vi "nirviRandomDataMultiElementFPGAFIFO.vi"(0 "Method":T1, 1 "Fifo":T2={"displayName"="", "hardwareName"="", "dataType"=enum."I16", "elementTypeDescriptor"=variant, "terminalTypeDescriptor"=variant, "requestedNumberOfElements"=2, "memoryType"=enum."Look-Up Table", "arbitrationForInterfaceA"=enum."Arbitrate if Multiple Requestors Only", "numberOfElementsPerRead"=1, "arbitrationForInterfaceB"=enum."Always Arbitrate", "numberOfElementsPerWrite"=1, "VI_Defined"=FALSE, "type"=enum."Target-Scoped", "initializationParameters"={"initialized"=FALSE, "VI_Path"=path "", "initialData"=variant}, "disableOnOverflow/Underflow"=FALSE, "interfaceConfiguration"=enum."Read A-Write B", "controlLogic"=enum."Slice Fabric", "actualNumberOfElements"=1027, "dramSelection"="", "dramMaxOustandingRequests"=0, "dramIncludeByteEnables"=FALSE, "dramGrantTime"=0, "fullEmulation"=FALSE, "memoryInMultipleClockDomains"=FALSE, "memoryLatency"=1} {"memoryLatency" items=["0", "1", "2", "3"]}, 3 "element in":variant, 5 "error in (no error)":errorcluster, 7 "Element Datatype":i32, 8 "In SCTL":bool, 9 "Input Valid?":bool, 11 "Timeout (ms)":i32, 13 "Ready for Output?":bool) -> (14 "element out":variant, 15 "Timed out":bool, 16 "Ready for Input":bool, 17 "count":u32, 18 "Output Valid":bool, 19 "error out":errorcluster)   [LabVIEW 2017]
uses:
  <vilib>/rvi/DataTransferAndStorage/Container/Common/niFpgaContainerState.ctl
  <vilib>/rvi/DataTransferAndStorage/Container/Common/niFpgaDataTypeControl.ctl
  <vilib>/rvi/DataTransferAndStorage/Container/Common/niFpgaContainerImplementationControl.ctl
  <vilib>/rvi/DataTransferAndStorage/Container/Common/niFpgaContainerArbitrationOptionsControl.ctl
  <vilib>/rvi/DataTransferAndStorage/Container/Common/niFpgaTransferTypeControl.ctl
  <vilib>/rvi/DataTransferAndStorage/Container/Common/niFpgaContainerInitializationParameters.ctl
  <vilib>/rvi/Memory/Memory_Types/niFpgaMemoryInterfaceConfiguration.ctl
  <vilib>/rvi/FIFO/Fifo_Types/niFpgaFifoControlLogicControl.ctl
  <vilib>/rvi/DataTransferAndStorage/Container/Common/niFpgaContainerMemoryLatencyControl.ctl
  <vilib>/rvi/DataTransferAndStorage/Container/Common/niFpgaContainerMethod.ctl
  <vilib>/rvi/interface/RandomDataEmulation/nirviQueueStoreOperation.ctl
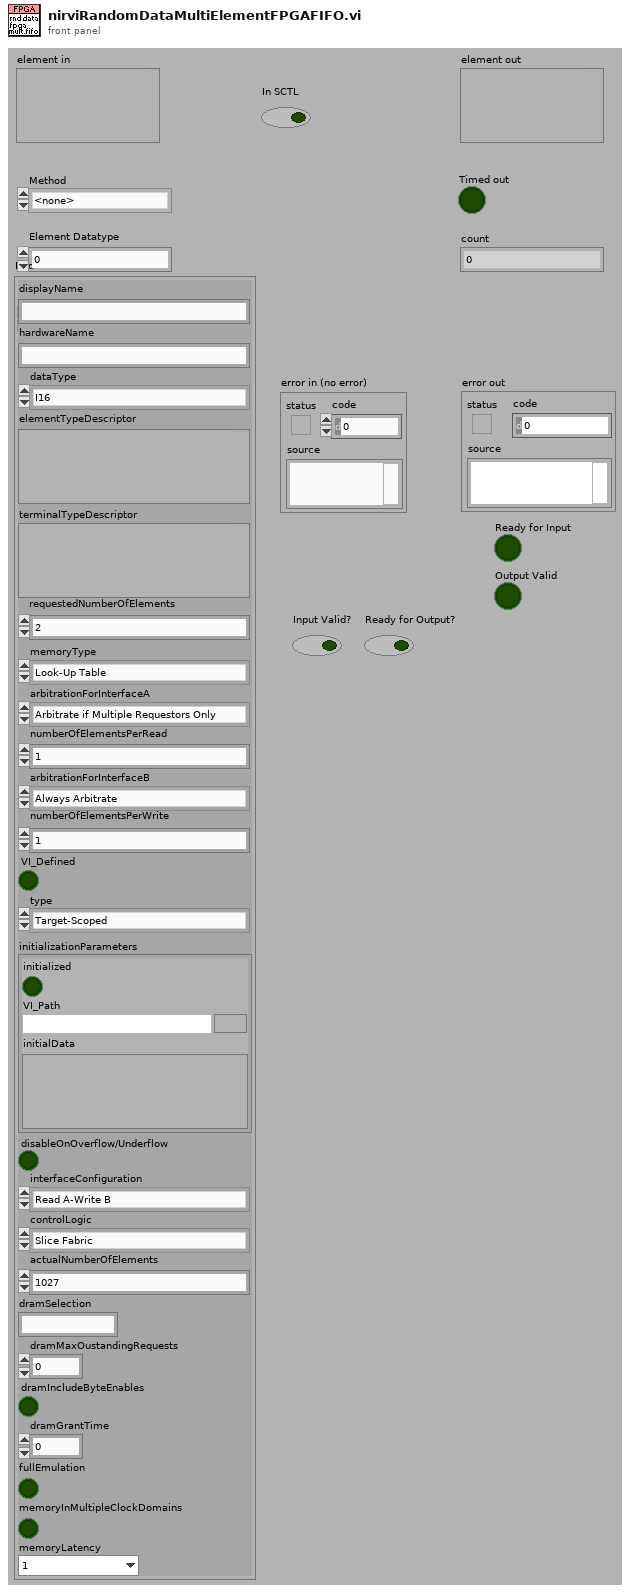
[diagram p1: front panel]
types:
  T1 = typedef "niFpgaContainerMethod.ctl" = enum16{"<none>", "write", "read", "clear", "getNumberOfElementsToWrite", "getNumberOfElementsToRead", "enable", "disable", "flushAndDisable", "getStreamState", "readA", "readB", "dramWrite", "dramWriteWithByteEnables", "dramRequestData", "dramRetrieveData", "readWithoutAcknowledge", "acknowledge", "writeUsingHandshaking", "readUsingHandshaking", "flush"}
  T2 = typedef "niFpgaContainerState.ctl" = cluster{"displayName":string, "hardwareName":string, "dataType":T3, "elementTypeDescriptor":variant, "terminalTypeDescriptor":variant, "requestedNumberOfElements":u32, "memoryType":T4, "arbitrationForInterfaceA":T5, "numberOfElementsPerRead":u32, "arbitrationForInterfaceB":T5, "numberOfElementsPerWrite":u32, "VI_Defined":bool, "type":T6, "initializationParameters":T7, "disableOnOverflow/Underflow":bool, "interfaceConfiguration":T8, "controlLogic":T9, "actualNumberOfElements":u32, "dramSelection":string, "dramMaxOustandingRequests":i32, "dramIncludeByteEnables":bool, "dramGrantTime":u32, "fullEmulation":bool, "memoryInMultipleClockDomains":bool, "memoryLatency":T10}
  T3 = typedef "niFpgaDataTypeControl.ctl" = enum32{"Boolean", "I8", "I16", "I32", "I64", "U8", "U16", "U32", "U64", "FXP", "CustomControl", "SGL"}
  T4 = typedef "niFpgaContainerImplementationControl.ctl" = enum16{"Flip-Flops", "Look-Up Table", "Block Memory", "DRAM"}
  T5 = typedef "niFpgaContainerArbitrationOptionsControl.ctl" = enum16{"Always Arbitrate", "Arbitrate if Multiple Requestors Only", "Never Arbitrate"}
  T6 = typedef "niFpgaTransferTypeControl.ctl" = enum16{"Target-Scoped", "Host to Target - DMA", "Target to Host - DMA", "Peer to Peer Reader", "Peer to Peer Writer", "Bidirectional"}
  T7 = typedef "niFpgaContainerInitializationParameters.ctl" = cluster{"initialized":bool, "VI_Path":path, "initialData":variant}
  T8 = typedef "niFpgaMemoryInterfaceConfiguration.ctl" = enum16{"Read A-Write B", "Read A-Read B"}
  T9 = typedef "niFpgaFifoControlLogicControl.ctl" = enum16{"Slice Fabric", "Target Optimal", "Built-in"}
  T10 = typedef "niFpgaContainerMemoryLatencyControl.ctl" = u16
  T11 = typedef "nirviQueueStoreOperation.ctl" = enum16{"Make New Queue", "Get Queue", "Resize Queue", "Close Queues", "Make New Lock", "Get Lock", "Get Host Fifo Size"}
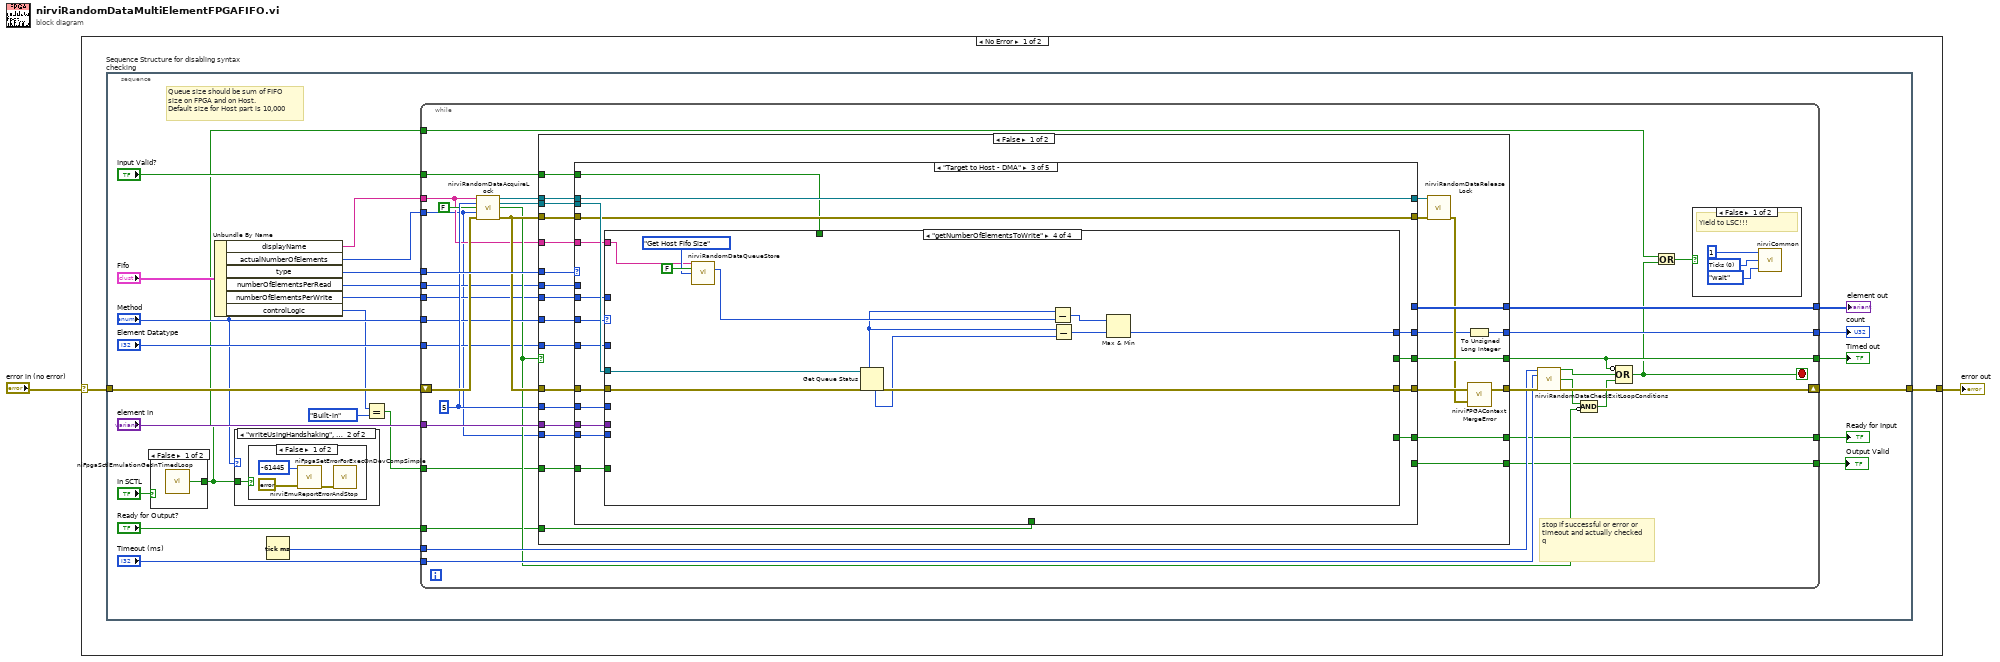
[diagram p0: block diagram]
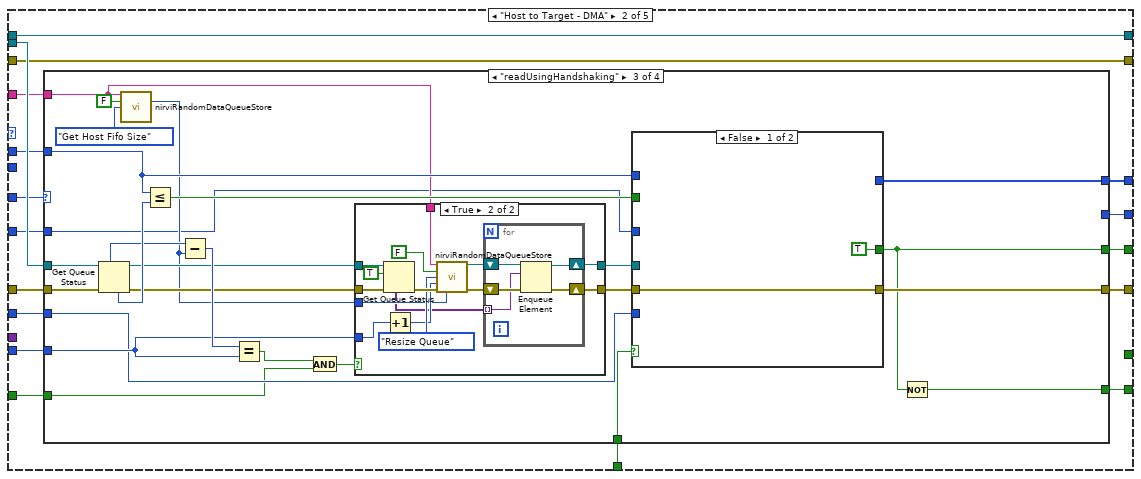
[diagram p7: hidden frame]
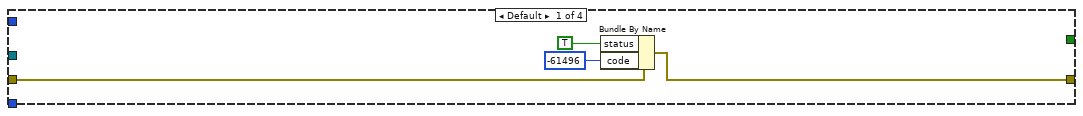
[diagram p8: hidden frame]
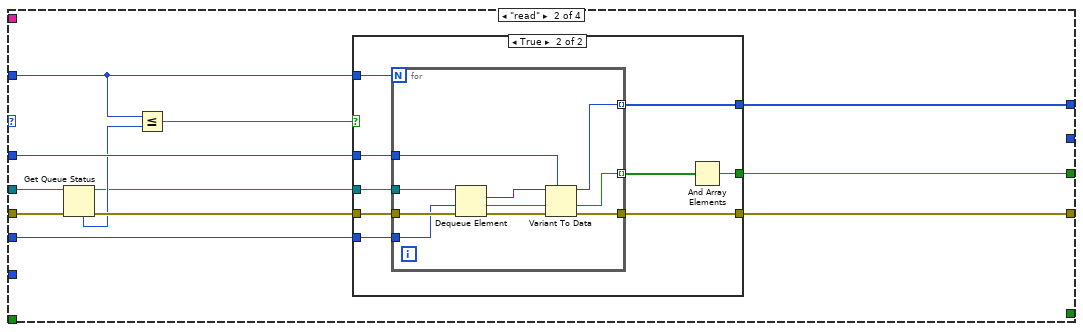
[diagram p9: hidden frame]
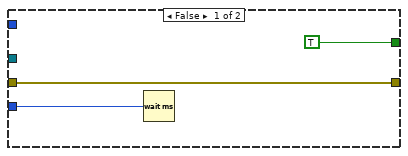
[diagram p10: hidden frame]
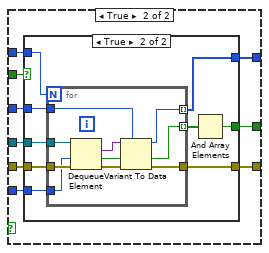
[diagram p11: hidden frame]
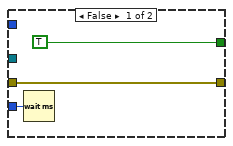
[diagram p12: hidden frame]
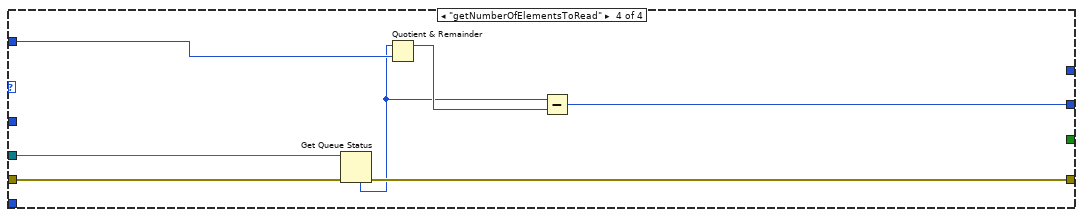
[diagram p14: hidden frame]
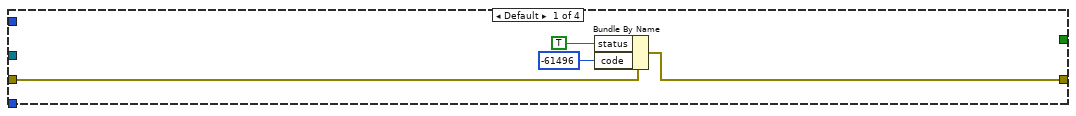
[diagram p15: hidden frame]
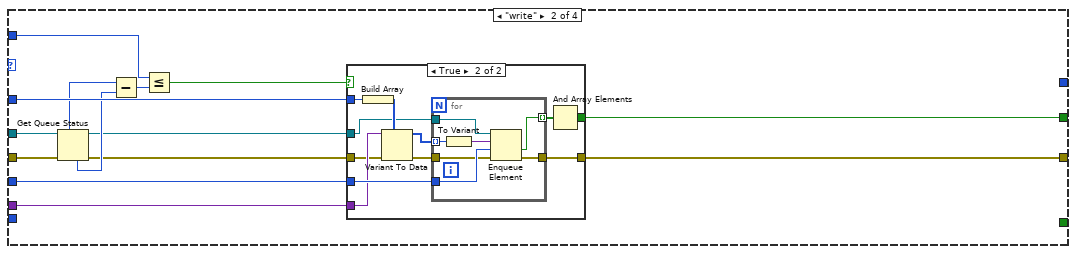
[diagram p16: hidden frame]
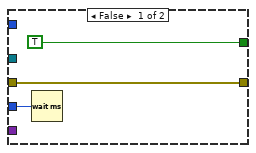
[diagram p17: hidden frame]
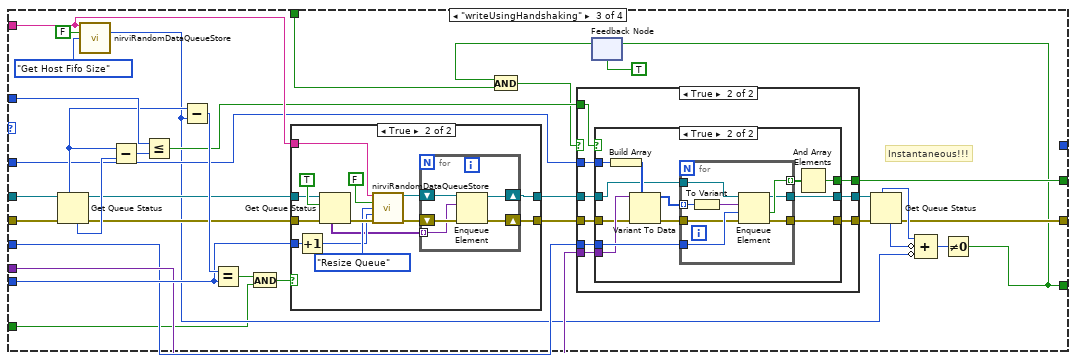
[diagram p18: hidden frame]
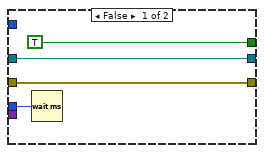
[diagram p20: hidden frame]
diagram:
  n1 = case shown="No Error" "error in (no error)" {
    selector: "error in (no error)" -> [w4 w413]
    tunnel: [w3 w413] -> w2
    frame No Error {
      n2 = stacked-sequence "Sequence Structure for disabling syntax checking" {
        tunnel: w4 -> [w15]
        tunnel: [w28] -> w3
        frame #0 {
          # "Queue size should be sum of FIFO\nsize on FPGA and on Host.\nDefault size for Host part is 10,000"
          n3 = case shown="False" "In SCTL" {
            selector: "In SCTL" -> [_ w31]
            tunnel: [w30 w31] -> w5
            frame False {
              n4 = call <vilib>:"niFpgaSctlEmulationGetInTimedLoop.vi"() -> ("x != 0?"=w30:bool)  [unwired: 15 in]
            }
            frame True {
            }
          }
          n5 = Unbundle By Name("Fifo") -> ("displayName"=w25:string, "actualNumberOfElements"=w23:u32, "type"=w22:T6, "numberOfElementsPerRead"=w18:u32, "numberOfElementsPerWrite"=w17:u32, "controlLogic"=w9:T9)
          n6 = case shown="\"writeUsingHandshaking\", \"readUsingHandshaking\"" "Method" {
            tunnel: w5 -> [_ w32]
            frame Default {
            }
            frame "writeUsingHandshaking", "readUsingHandshaking" {
              n7 = case shown="False" w32 {
                frame False {
                  n8 = call <vilib>:"niFpgaSetErrorForExecOnDevCompSimple.vi"("error code"=-61445, "error in"=errorcluster {"status"=FALSE, "code"=0, "source"=""}) -> ("error out"=w35:errorcluster)  [unwired: 13 in]
                  n9 = call <vilib>:"nirviEmuReportErrorAndStop.vi"("error to report"=w35) -> ()  [unwired: 1 in, 14 out]
                }
                frame True {
                }
              }
            }
          }
          n10 = Tick Count (ms)() -> (millisecond timer value=w27:u32)
          n11 = Equal?(x=w9, y=niFpgaFifoControlLogicControl."Built-in") -> (x = y?=w7:bool)
          n12 = while {
            tunnel: w22 -> [w66]
            tunnel: "element in" -> [w68]
            tunnel: "Timeout (ms)" -> [w62]
            tunnel: [w67] -> w26
            tunnel: [w54] -> w20
            tunnel: w27 -> [w63]
            tunnel: w25 -> [w45]
            shift-right: [w65] -> w28
            shift-left: w15 -> [w61]
            tunnel: w23 -> [w44]
            tunnel: "Method" -> [w55]
            tunnel: [w53] -> w19
            tunnel: "Element Datatype" -> [w48]
            tunnel: w18 -> [w47]
            tunnel: w17 -> [w46]
            tunnel: "Ready for Output?" -> [w43]
            tunnel: [w42] -> w12
            tunnel: "Input Valid?" -> [w41]
            tunnel: [w40] -> w10
            tunnel: w7 -> [w39]
            tunnel: w5 -> [w37]
            stop <- w38 stop-if-true
            w59 = 5 ("ms timeout (-1)")
            # "stop if successful or error or \ntimeout and actually checked q"
            n13 = call <vilib>:"nirviRandomDataAcquireLock.vi"("name"=w45, "ms timeout (-1)"=w59, "Host?"=FALSE, "fpga fifo size"=w44, "error in (no error)"=w61) -> ("lock out"=w60:refnum<queue>, "queue out"=w57:refnum<queue>, "timed out"=w52:bool, "error out"=w56:errorcluster)  [unwired: 7 out]
            n14 = case shown="False" w52 {
              selector: w52 -> [_ w412]
              tunnel: w68 -> [w84 _]
              tunnel: w59 -> [w98 _]
              tunnel: [w97 _] -> w67
              tunnel: [w93 w411] -> w64
              tunnel: [w96 w412] -> w54
              tunnel: w66 -> [w95 _]
              tunnel: w56 -> [w90 w411]
              tunnel: w60 -> [w85 _]
              tunnel: w57 -> [w91 _]
              tunnel: w56 -> [w88 _]
              tunnel: w55 -> [w87 _]
              tunnel: [w82 _] -> w53
              tunnel: w48 -> [w81 _]
              tunnel: w47 -> [w80 _]
              tunnel: w46 -> [w79 _]
              tunnel: w45 -> [w78 _]
              tunnel: w44 -> [w77 _]
              tunnel: w43 -> [w76 _]
              tunnel: [w75 _] -> w42
              tunnel: w41 -> [w74 _]
              tunnel: [w73 _] -> w40
              tunnel: w39 -> [w72 _]
              frame False {
                n15 = case shown="\"Target to Host - DMA\"" w95 {
                  tunnel: w98 -> [_ w117 w258 _ _]
                  tunnel: [_ w116 w256 _ _] -> w96
                  tunnel: [w101 w118 w259 w404 w405] -> w94
                  tunnel: [_ w108 _ _ _] -> w97
                  tunnel: w84 -> [_ _ w257 _ _]
                  tunnel: w90 -> [w101 w115 w255 w404 w406]
                  tunnel: w91 -> [_ w114 w254 _ _]
                  tunnel: [w100 w113 w253 w403 w407] -> w89
                  tunnel: w88 -> [w100 w113 w253 w403 w407]
                  tunnel: w87 -> [_ w111 w251 _ _]
                  tunnel: [w99 w112 w252 w402 w410] -> w86
                  tunnel: w85 -> [w99 w112 w252 w402 w410]
                  tunnel: [_ w110 w243 _ _] -> w83
                  tunnel: w81 -> [_ w109 w250 _ _]
                  tunnel: w80 -> [_ w107 _ _ _]
                  tunnel: w79 -> [_ _ w249 _ _]
                  tunnel: w78 -> [_ w106 w248 _ _]
                  tunnel: w77 -> [_ w105 w247 _ _]
                  tunnel: w76 -> [_ w104 _ _ _]
                  tunnel: [_ w103 _ _ _] -> w75
                  tunnel: w74 -> [_ _ w246 _ _]
                  tunnel: [_ _ w245 _ _] -> w73
                  tunnel: w72 -> [_ w102 w244 _ _]
                  frame "Target-Scoped" {
                    # "Not a DMA FIFO"
                  }
                  frame "Host to Target - DMA" {
                    n16 = case shown="\"readUsingHandshaking\"" w111 {
                      tunnel: [w119 w134 w181 w242] -> w118
                      tunnel: w117 -> [_ w132 w164 _]
                      tunnel: [_ w131 w161 _] -> w116
                      tunnel: w115 -> [w120 w129 w179 w240]
                      tunnel: w114 -> [_ w125 w176 w241]
                      tunnel: [_ _ _ w236] -> w110
                      tunnel: w109 -> [_ w133 w159 _]
                      tunnel: [_ w130 w180 _] -> w108
                      tunnel: w107 -> [_ w127 w178 w238]
                      tunnel: w106 -> [_ _ w170 _]
                      tunnel: w105 -> [_ _ w166 _]
                      tunnel: w104 -> [_ _ w162 _]
                      tunnel: [_ _ w160 _] -> w103
                      tunnel: w102 -> [_ _ w157 _]
                      frame Default {
                        n17 = Bundle By Name(cluster=w120, "status"=TRUE, "code"=-61496) -> (w119:errorcluster)
                      }
                      frame "read" {
                        n18 = Get Queue Status(queue=w125, error in (no error)=w129) -> (queue out=w124:refnum<queue>, error out=w128:errorcluster, # elements in queue=w126:i32)  [unwired: 1 in, 5 out]
                        n19 = Less Or Equal?(x=w127, y=w126) -> (x <= y?=w123:bool)
                        n20 = case shown="True" w123 {
                          tunnel: [w137 w146] -> w134
                          tunnel: w133 -> [_ w145]
                          tunnel: w132 -> [w135 w144]
                          tunnel: [TRUE ("timed out?") w138] -> w131
                          tunnel: [_ w143] -> w130
                          tunnel: w128 -> [w137 w142]
                          tunnel: w127 -> [_ w141]
                          tunnel: w124 -> [_ w140]
                          frame False {
                            n21 = Wait (ms)(milliseconds to wait=w135) -> ()  [unwired: 1 out]
                          }
                          frame True {
                            n22 = for {
                              N: w141 -> [_]
                              tunnel: [w155] -> w139 mode=indexing
                              tunnel: [w151] -> w146
                              tunnel: [w149] -> w143 mode=indexing
                              tunnel: w142 -> [w154]
                              tunnel: w145 -> [w150]
                              tunnel: w144 -> [w148]
                              tunnel: w140 -> [w147]
                              n23 = Dequeue Element(queue=w147, timeout in ms (-1)=w148, error in (no error)=w154) -> (element=w153:variant, timed out?=w155:bool, error out=w152:errorcluster)  [unwired: 1 out]
                              n24 = Variant To Data(error in=w152, type=w150, Variant=w153) -> (data=w149:i32, error out=w151:errorcluster)
                            }
                            n25 = And Array Elements(Boolean array=w139) -> (logical AND=w138:bool)
                          }
                        }
                      }
                      frame "readUsingHandshaking" {
                        n26 = Get Queue Status(queue=w176, error in (no error)=w179) -> (queue out=w169:refnum<queue>, max queue size=w172:i32, error out=w167:errorcluster, # elements in queue=w177:i32)  [unwired: 1 in, 4 out]
                        n27 = call <vilib>:"nirviRandomDataQueueStore.vi"("queue name"=w170, "Host?"=FALSE, "queue operation"=nirviQueueStoreOperation."Get Host Fifo Size") -> ("host fifo size out"=w165:u32)  [unwired: 9 in, 3 out]
                        n28 = Less Or Equal?(x=w178, y=w177) -> (x <= y?=w175:bool)
                        n29 = Subtract(x=w172, y=w165) -> (x-y=w171:u32)
                        n30 = Equal?(x=w171, y=w166) -> (x = y?=w158:bool)
                        n31 = And(x=w158, y=w157) -> (x .and. y?=w156:bool)
                        n32 = case shown="True" w156 {
                          tunnel: w167 -> [w214 w230]
                          tunnel: w169 -> [w215 w229]
                          tunnel: w170 -> [_ w226]
                          tunnel: w166 -> [_ w223]
                          tunnel: w165 -> [_ w221]
                          tunnel: [w215 w218] -> w168
                          tunnel: [w214 w216] -> w163
                          frame False {
                          }
                          frame True {
                            n33 = Get Queue Status(queue=w229, return elements? (F)=TRUE, error in (no error)=w230) -> (error out=w227:errorcluster, elements=w220:variant[])  [unwired: 6 out]
                            n34 = Increment(x=w223) -> (x+1=w222:u32)
                            n35 = call <vilib>:"nirviRandomDataQueueStore.vi"("queue name"=w226, "Host?"=FALSE, "queue operation"=nirviQueueStoreOperation."Resize Queue", "fpga fifo size"=w222, "error in (no error)"=w227, "host fifo size"=w221) -> ("queue out"=w219:refnum<queue>, "error out"=w217:errorcluster)  [unwired: 6 in, 2 out]
                            n36 = for {
                              tunnel: w220 -> [w233] mode=indexing
                              shift-right: [w231] -> w218
                              shift-left: w219 -> [w234]
                              shift-right: [w232] -> w216
                              shift-left: w217 -> [w235]
                              n37 = Enqueue Element(queue=w234, element=w233, error in (no error)=w235) -> (queue out=w231:refnum<queue>, error out=w232:errorcluster)  [unwired: 1 in, 1 out]
                            }
                          }
                        }
                        n38 = case shown="False" w162 {
                          tunnel: [w183 w192] -> w181
                          tunnel: [TRUE ("timed out?") w191] -> w161
                          tunnel: [_ w190] -> w180
                          tunnel: w178 -> [_ w189]
                          tunnel: w175 -> [_ w188]
                          tunnel: w168 -> [_ w187]
                          tunnel: w164 -> [_ w186]
                          tunnel: w163 -> [w183 w185]
                          tunnel: w159 -> [_ w184]
                          frame False {
                          }
                          frame True {
                            n39 = case shown="True" w188 {
                              tunnel: [w195 w204] -> w192
                              tunnel: w184 -> [_ w203]
                              tunnel: w186 -> [w193 w202]
                              tunnel: [TRUE ("timed out?") w197] -> w191
                              tunnel: [_ w201] -> w190
                              tunnel: w185 -> [w195 w200]
                              tunnel: w189 -> [_ w196]
                              tunnel: w187 -> [_ w199]
                              frame False {
                                n40 = Wait (ms)(milliseconds to wait=w193) -> ()  [unwired: 1 out]
                              }
                              frame True {
                                n41 = for {
                                N: w196 -> [_]
                                tunnel: [w213] -> w198 mode=indexing
                                tunnel: [w209] -> w204
                                tunnel: [w207] -> w201 mode=indexing
                                tunnel: w200 -> [w212]
                                tunnel: w203 -> [w208]
                                tunnel: w202 -> [w206]
                                tunnel: w199 -> [w205]
                                n42 = Dequeue Element(queue=w205, timeout in ms (-1)=w206, error in (no error)=w212) -> (element=w211:variant, timed out?=w213:bool, error out=w210:errorcluster)  [unwired: 1 out]
                                n43 = Variant To Data(error in=w210, type=w208, Variant=w211) -> (data=w207:i32, error out=w209:errorcluster)
                                }
                                n44 = And Array Elements(Boolean array=w198) -> (logical AND=w197:bool)
                              }
                            }
                          }
                        }
                        n45 = Not(x=w161) -> (.not. x?=w160:bool)
                      }
                      frame "getNumberOfElementsToRead" {
                        n46 = Get Queue Status(queue=w241, error in (no error)=w240) -> (error out=w242:errorcluster, # elements in queue=w237:i32)  [unwired: 1 in, 6 out]
                        n47 = Quotient & Remainder(x=w237, y=w238) -> (x-y*floor(x/y)=w239:u32)  [unwired: 1 out]
                        n48 = Subtract(x=w237, y=w239) -> (x-y=w236:u32)
                      }
                    }
                  }
                  frame "Target to Host - DMA" {
                    n49 = case shown="\"getNumberOfElementsToWrite\"" w251 {
                      tunnel: [w260 w277 w303 w399] -> w259
                      tunnel: w258 -> [_ w276 w317 _]
                      tunnel: w257 -> [_ w273 w318 _]
                      tunnel: [_ w274 w333 _] -> w256
                      tunnel: w255 -> [w261 w270 w331 w400]
                      tunnel: w254 -> [_ w268 w330 w401]
                      tunnel: w250 -> [_ w275 w315 _]
                      tunnel: w249 -> [_ w265 w328 _]
                      tunnel: w248 -> [_ _ w323 w396]
                      tunnel: w247 -> [_ _ w320 _]
                      tunnel: w246 -> [_ _ w311 _]
                      tunnel: [_ _ w299 _] -> w245
                      tunnel: w244 -> [_ _ w300 _]
                      tunnel: [_ _ _ w393] -> w243
                      frame Default {
                        n50 = Bundle By Name(cluster=w261, "status"=TRUE, "code"=-61496) -> (w260:errorcluster)
                      }
                      frame "write" {
                        n51 = Get Queue Status(queue=w268, error in (no error)=w270) -> (queue out=w267:refnum<queue>, max queue size=w272:i32, error out=w269:errorcluster, # elements in queue=w271:i32)  [unwired: 1 in, 4 out]
                        n52 = Subtract(x=w272, y=w271) -> (x-y=w266:i32)
                        n53 = Less Or Equal?(x=w265, y=w266) -> (x <= y?=w264:bool)
                        n54 = case shown="True" w264 {
                          tunnel: [w279 w291] -> w277
                          tunnel: w276 -> [w278 w290]
                          tunnel: w275 -> [_ w287]
                          tunnel: [TRUE w284] -> w274
                          tunnel: w273 -> [_ w283]
                          tunnel: w269 -> [w279 w282]
                          tunnel: w267 -> [_ w281]
                          frame False {
                            n55 = Wait (ms)(milliseconds to wait=w278) -> ()  [unwired: 1 out]
                          }
                          frame True {
                            n56 = Build Array(w287) -> (w285:i32[])
                            n57 = Variant To Data(error in=w282, type=w285, Variant=w283) -> (data=w286:i32[], error out=w288:errorcluster)
                            n58 = for {
                              tunnel: [w298] -> w291
                              tunnel: w290 -> [w297]
                              tunnel: [w296] -> w289 mode=indexing
                              tunnel: w281 -> [w295]
                              tunnel: w288 -> [w294]
                              tunnel: w286 -> [w293] mode=indexing
                              n59 = To Variant(anything=w293) -> (Variant=w292:variant)
                              n60 = Enqueue Element(queue=w295, element=w292, timeout in ms (-1)=w297, error in (no error)=w294) -> (timed out?=w296:bool, error out=w298:errorcluster)  [unwired: 1 out]
                            }
                            n61 = And Array Elements(Boolean array=w289) -> (logical AND=w284:bool)
                          }
                        }
                      }
                      frame "writeUsingHandshaking" {
                        # "Instantaneous!!!"
                        n62 = Get Queue Status(queue=w330, error in (no error)=w331) -> (queue out=w322:refnum<queue>, max queue size=w325:i32, error out=w321:errorcluster, # elements in queue=w332:i32)  [unwired: 1 in, 4 out]
                        n63 = call <vilib>:"nirviRandomDataQueueStore.vi"("queue name"=w323, "Host?"=FALSE, "queue operation"=nirviQueueStoreOperation."Get Host Fifo Size") -> ("host fifo size out"=w306:u32)  [unwired: 9 in, 3 out]
                        n64 = Subtract(x=w325, y=w332) -> (x-y=w329:i32)
                        n65 = Less Or Equal?(x=w328, y=w329) -> (x <= y?=w313:bool)
                        n66 = Subtract(x=w325, y=w306) -> (x-y=w324:u32)
                        n67 = Equal?(x=w324, y=w320) -> (x = y?=w302:bool)
                        n68 = And(x=w302, y=w300) -> (x .and. y?=w301:bool)
                        n69 = case shown="True" w301 {
                          tunnel: w321 -> [w370 w384]
                          tunnel: [w369 w376] -> w316
                          tunnel: [w370 w374] -> w319
                          tunnel: w322 -> [w369 w373]
                          tunnel: w320 -> [_ w372]
                          tunnel: w323 -> [_ w371]
                          frame False {
                          }
                          frame True {
                            n70 = Increment(x=w372) -> (x+1=w379:u32)
                            n71 = Get Queue Status(queue=w373, return elements? (F)=TRUE, error in (no error)=w384) -> (error out=w382:errorcluster, elements=w378:variant[])  [unwired: 6 out]
                            n72 = call <vilib>:"nirviRandomDataQueueStore.vi"("queue name"=w371, "Host?"=FALSE, "queue operation"=nirviQueueStoreOperation."Resize Queue", "fpga fifo size"=w379, "error in (no error)"=w382) -> ("queue out"=w377:refnum<queue>, "error out"=w375:errorcluster)  [unwired: 7 in, 2 out]
                            n73 = for {
                              tunnel: w378 -> [w387] mode=indexing
                              shift-right: [w385] -> w376
                              shift-left: w377 -> [w388]
                              shift-right: [w386] -> w374
                              shift-left: w375 -> [w389]
                              n74 = Enqueue Element(queue=w388, element=w387, error in (no error)=w389) -> (queue out=w385:refnum<queue>, error out=w386:errorcluster)  [unwired: 1 in, 1 out]
                            }
                          }
                        }
                        n75 = feedback #1(TRUE) -> (w312:bool)
                        n76 = And(x=w312, y=w311) -> (x .and. y?=w304:bool)
                        n77 = case shown="True" w304 {
                          tunnel: [w335 w344] -> w310
                          tunnel: [_ w343] -> w333
                          tunnel: w319 -> [w335 w342]
                          tunnel: w318 -> [_ w341]
                          tunnel: w317 -> [_ w340]
                          tunnel: w316 -> [w334 w339]
                          tunnel: w315 -> [_ w338]
                          tunnel: w313 -> [_ w337]
                          tunnel: [w334 w336] -> w309
                          frame False {
                          }
                          frame True {
                            n78 = case shown="True" w337 {
                              tunnel: [w347 w360] -> w344
                              tunnel: w340 -> [w346 w359]
                              tunnel: w338 -> [_ w356]
                              tunnel: [TRUE w353] -> w343
                              tunnel: w341 -> [_ w352]
                              tunnel: w342 -> [w347 w351]
                              tunnel: w339 -> [w345 w350]
                              tunnel: [w345 w349] -> w336
                              frame False {
                                n79 = Wait (ms)(milliseconds to wait=w346) -> ()  [unwired: 1 out]
                              }
                              frame True {
                                n80 = Build Array(w356) -> (w354:i32[])
                                n81 = Variant To Data(error in=w351, type=w354, Variant=w352) -> (data=w355:i32[], error out=w357:errorcluster)
                                n82 = for {
                                tunnel: [w368] -> w360
                                tunnel: w359 -> [w367]
                                tunnel: [w366] -> w358 mode=indexing
                                tunnel: w350 -> [w365]
                                tunnel: w357 -> [w364]
                                tunnel: w355 -> [w363] mode=indexing
                                tunnel: [w361] -> w349
                                n83 = To Variant(anything=w363) -> (Variant=w362:variant)
                                n84 = Enqueue Element(queue=w365, element=w362, timeout in ms (-1)=w367, error in (no error)=w364) -> (queue out=w361:refnum<queue>, timed out?=w366:bool, error out=w368:errorcluster)
                                }
                                n85 = And Array Elements(Boolean array=w358) -> (logical AND=w353:bool)
                              }
                            }
                          }
                        }
                        n86 = Get Queue Status(queue=w309, error in (no error)=w310) -> (max queue size=w308:i32, error out=w303:errorcluster, # elements in queue=w307:i32)  [unwired: 1 in, 5 out]
                        n87 = Compound Arithmetic op=ADD(w308, invert w307, invert w306) -> (w305:u32)
                        n88 = Not Equal To 0?(x=w305) -> (x != 0?=w299:bool)
                        n89 = feedback-in #1(w299) -> ()
                      }
                      frame "getNumberOfElementsToWrite" {
                        n90 = call <vilib>:"nirviRandomDataQueueStore.vi"("queue name"=w396, "Host?"=FALSE, "queue operation"=nirviQueueStoreOperation."Get Host Fifo Size") -> ("host fifo size out"=w392:u32)  [unwired: 9 in, 3 out]
                        n91 = Get Queue Status(queue=w401, error in (no error)=w400) -> (max queue size=w391:i32, error out=w399:errorcluster, # elements in queue=w390:i32)  [unwired: 1 in, 5 out]
                        n92 = Subtract(x=w391, y=w392) -> (x-y=w394:u32)
                        n93 = Subtract(x=w391, y=w390) -> (x-y=w395:i32)
                        n94 = Max & Min(x=w394, y=w395) -> (min(x,y)=w393:u32)  [unwired: 1 out]
                      }
                    }
                  }
                  frame "Peer to Peer Reader", "Peer to Peer Writer" {
                    # "No emulation support"
                  }
                  frame "Bidirectional" {
                    # "Other methods aren't supported by FIFOs."
                    n95 = Bundle By Name(cluster=w406, "status"=TRUE, "code"=-61496) -> (w405:errorcluster)
                  }
                }
                n96 = call <vilib>:"nirviRandomDataReleaseLock.vi"("lock in"=w86, "error in (no error)"=w89) -> ("error out"=w92:errorcluster)  [unwired: 13 out]
                n97 = To Unsigned Long Integer(number=w83) -> (unsigned 32bit integer=w82:u32)
                n98 = call <vilib>:"nirviFPGAContextMergeError.vi"("error 2"=w92, "error 1"=w94) -> ("error out"=w93:errorcluster)
              }
              frame True {
              }
            }
            n99 = call <vilib>:"nirviRandomDataCheckExitLoopConditions.vi"("Start Time"=w63, "Timeout (ms)"=w62, "error in (no error)"=w64) -> ("Error Occurred"=w49:bool, "Timed Out"=w51:bool, "error out"=w65:errorcluster)  [unwired: 10 out]
            n100 = Compound Arithmetic op=AND(w51, invert w52) -> (w50:bool)
            n101 = Compound Arithmetic op=OR(invert w54, w49, w50) -> (w38:bool)
            n102 = Or(x=w37, y=w38) -> (x .or. y?=w36:bool)
            n103 = case shown="False" w36 {
              frame False {
                w70 = u16 0 items=["Ticks", "µSec", "mSec"] ("Counter Units")
                # "Yield to LSC!!!"
                n104 = call <vilib>:"nirviCommon.vi"("Action"=enum16{"wait", "wait multiple", "tick count"}."wait", "Counter Units"=w70, "Count(uSec)"=u32 1) -> ()  [unwired: 1 out]
              }
              frame True {
              }
            }
          }
          "element out" <- w26
          "Timed out" <- w20
          "count" <- w19
          "Ready for Input" <- w10
          "Output Valid" <- w12
        }
      }
    }
    frame Error {
    }
  }
  "error out" <- w2
